vi "Set Up Worldmap Graph.vi"(8 "error in (no error)":errorcluster, 10 "Path to PNG file":path, 11 "XYGraph Refnum":refnum<vi>) -> (0 "error out":errorcluster)   [LabVIEW 2018]
doc: "Sets up the properties of an XY plot to display thePNG file as background and use latitude/longitude coordinates."
uses:
  <vilib>/Utility/miscctls.llb/LVMajorAndMinorColorsTypeDef.ctl
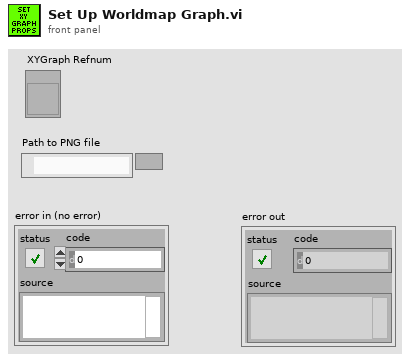
[diagram p1: front panel]
types:
  T1 = typedef "LVMajorAndMinorColorsTypeDef.ctl" = cluster{"Major Color":u32, "Minor Color":u32}
  T2 = typedef "imagedata.ctl" = cluster{"image type":i32, "image depth":i32, "image":u8[], "mask":u8[], "colors":u32[], "Rectangle":cluster{"left":i16, "top":i16, "right":i16, "bottom":i16}}
  T3 = cluster{"left":i16, "top":i16, "right":i16, "bottom":i16}
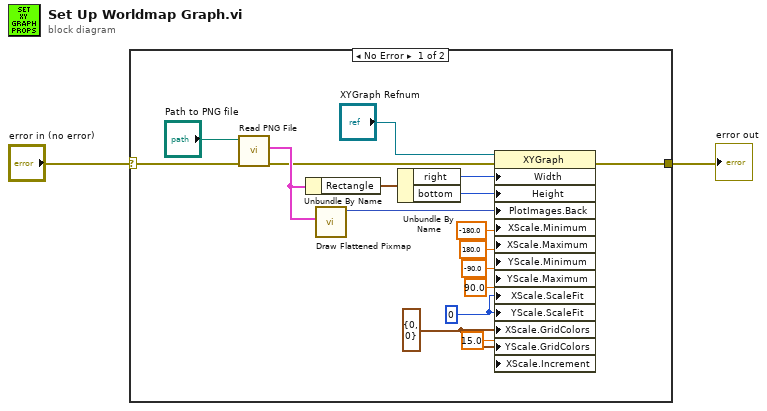
[diagram p0: block diagram]
diagram:
  n1 = case shown="No Error" "error in (no error)" {
    selector: "error in (no error)" -> [w5 w20]
    tunnel: [w4 w20] -> w1
    frame No Error {
      w10 = T1 {"Major Color"=0, "Minor Color"=0} ("X Scale.Grid Colors")
      w11 = u8 0 ("Y Scale.Scale Fit")
      n2 = call <vilib>:"Read PNG File.vi"("error in (no error)"=w5, "path to PNG file"="Path to PNG file") -> ("error out"=w8:errorcluster, "image data"=w16:T2)  [unwired: 7 in, 1 out]
      n3 = Unbundle By Name(w16) -> ("Rectangle"=w19:T3)
      n4 = call <vilib>:"Draw Flattened Pixmap.vi"("image data"=w16) -> ("new picture"=w9:picture)  [unwired: 8 in]
      n5 = Unbundle By Name(w19) -> ("right"=w18:i16, "bottom"=w17:i16)
      n6 = property on="Property Node" class="XYGraph"(reference="XYGraph Refnum", error in=w8, "Width"=w18, "Height"=w17, "PlotImages.Back"=w9, "XScale.Minimum"=-180.0 ("X Scale.Range:Minimum"), "XScale.Maximum"=180.0 ("X Scale.Range:Maximum"), "YScale.Minimum"=-90.0 ("Y Scale.Range:Minimum"), "YScale.Maximum"=90.0 ("Y Scale.Range:Maximum"), "XScale.ScaleFit"=w11, "YScale.ScaleFit"=w11, "XScale.GridColors"=w10, "YScale.GridColors"=w10, "XScale.Increment"=15.0 ("X Scale.Range:Increment")) -> (error out=w4:errorcluster)  [unwired: 1 out]
    }
    frame Error {
    }
  }
  "error out" <- w1
